vi "Send GUI Update Displays.vi"(8 "error in":errorcluster) -> (0 "error out":errorcluster)   [LabVIEW 2013]
doc: "Sends a message to the main loop to update the image displays"
uses:
  MsgQ Loops enum.ctl
  Main MsgQ.lvlib
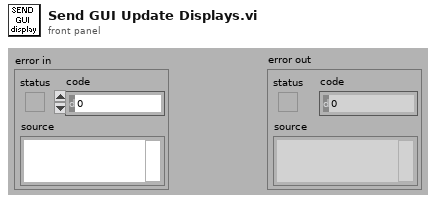
[diagram p1: front panel]
types:
  T1 = typedef "Main MsgQ.lvlib/MsgQ Loops enum.ctl" = enum16{"User Interface", "Image Acq"}
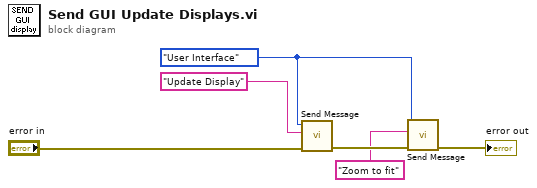
[diagram p0: block diagram]
diagram:
  w4 = MsgQ_Loops_enum."User Interface" ("Send to MsgQ")
  n1 = call "Send Message.vi"("error in (no error)"="error in", "Message String"="Update Display", "Send to MsgQ"=w4) -> ("error out"=w3:errorcluster)  [unwired: 1 in, 7 out]
  n2 = call "Send Message.vi"("error in (no error)"=w3, "Message String"="Zoom to fit", "Send to MsgQ"=w4) -> ("error out"=→"error out":errorcluster)  [unwired: 1 in, 7 out]
